vi "Main-OpenByFileVersionLabVIEW.vi"() -> ()   [LabVIEW 2017]
uses:
  States.ctl
  <vilib>/Utility/sysdir.llb/System Directory Type.ctl
  C:/Windows/System32/user32.dll
panel:
  in  "Simulation File Path":path
  in  "Simulation?":bool
  out "File Name & Version":string
  # "File :\nLabVIEW Version :\n\n\nAuthor :\nWebsite :"
  # "Ajay\nhttps://www.digiajay.com/"
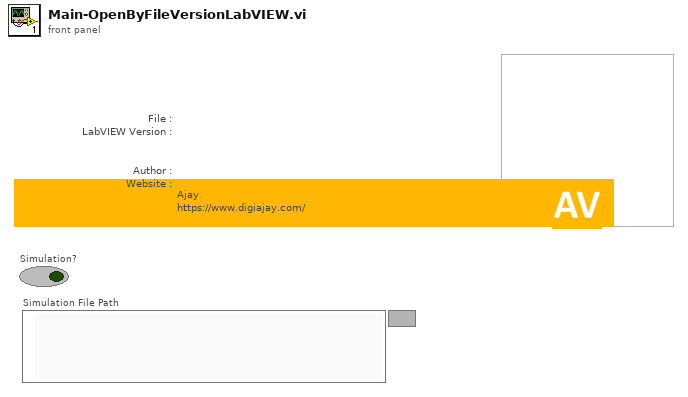
[diagram p1: front panel]
types:
  T1 = cluster{"File Path":path, "File LV Version":string, "File LV Exe Path":path, "Latest LV Exe Path":path, "Timeout Counter":i32, "NI Apps Folder":path, "Open x64 Bit?":bool, "Process Handle":refnum<k24>}
  T2 = typedef "States.ctl" = enum16{"Show FP", "Get LV Version & Path", "Update FP", "Get NI App Folder", "Get File LV Exe Path", "Get Latest LV Exe Path", "Open File Version LV", "Poll", "Exit"}
  T3 = enum32{"Invalid", "Standard", "Closed", "Hidden", "Minimized", "Maximized"}
  T4 = typedef "System Directory Type.ctl" = i32
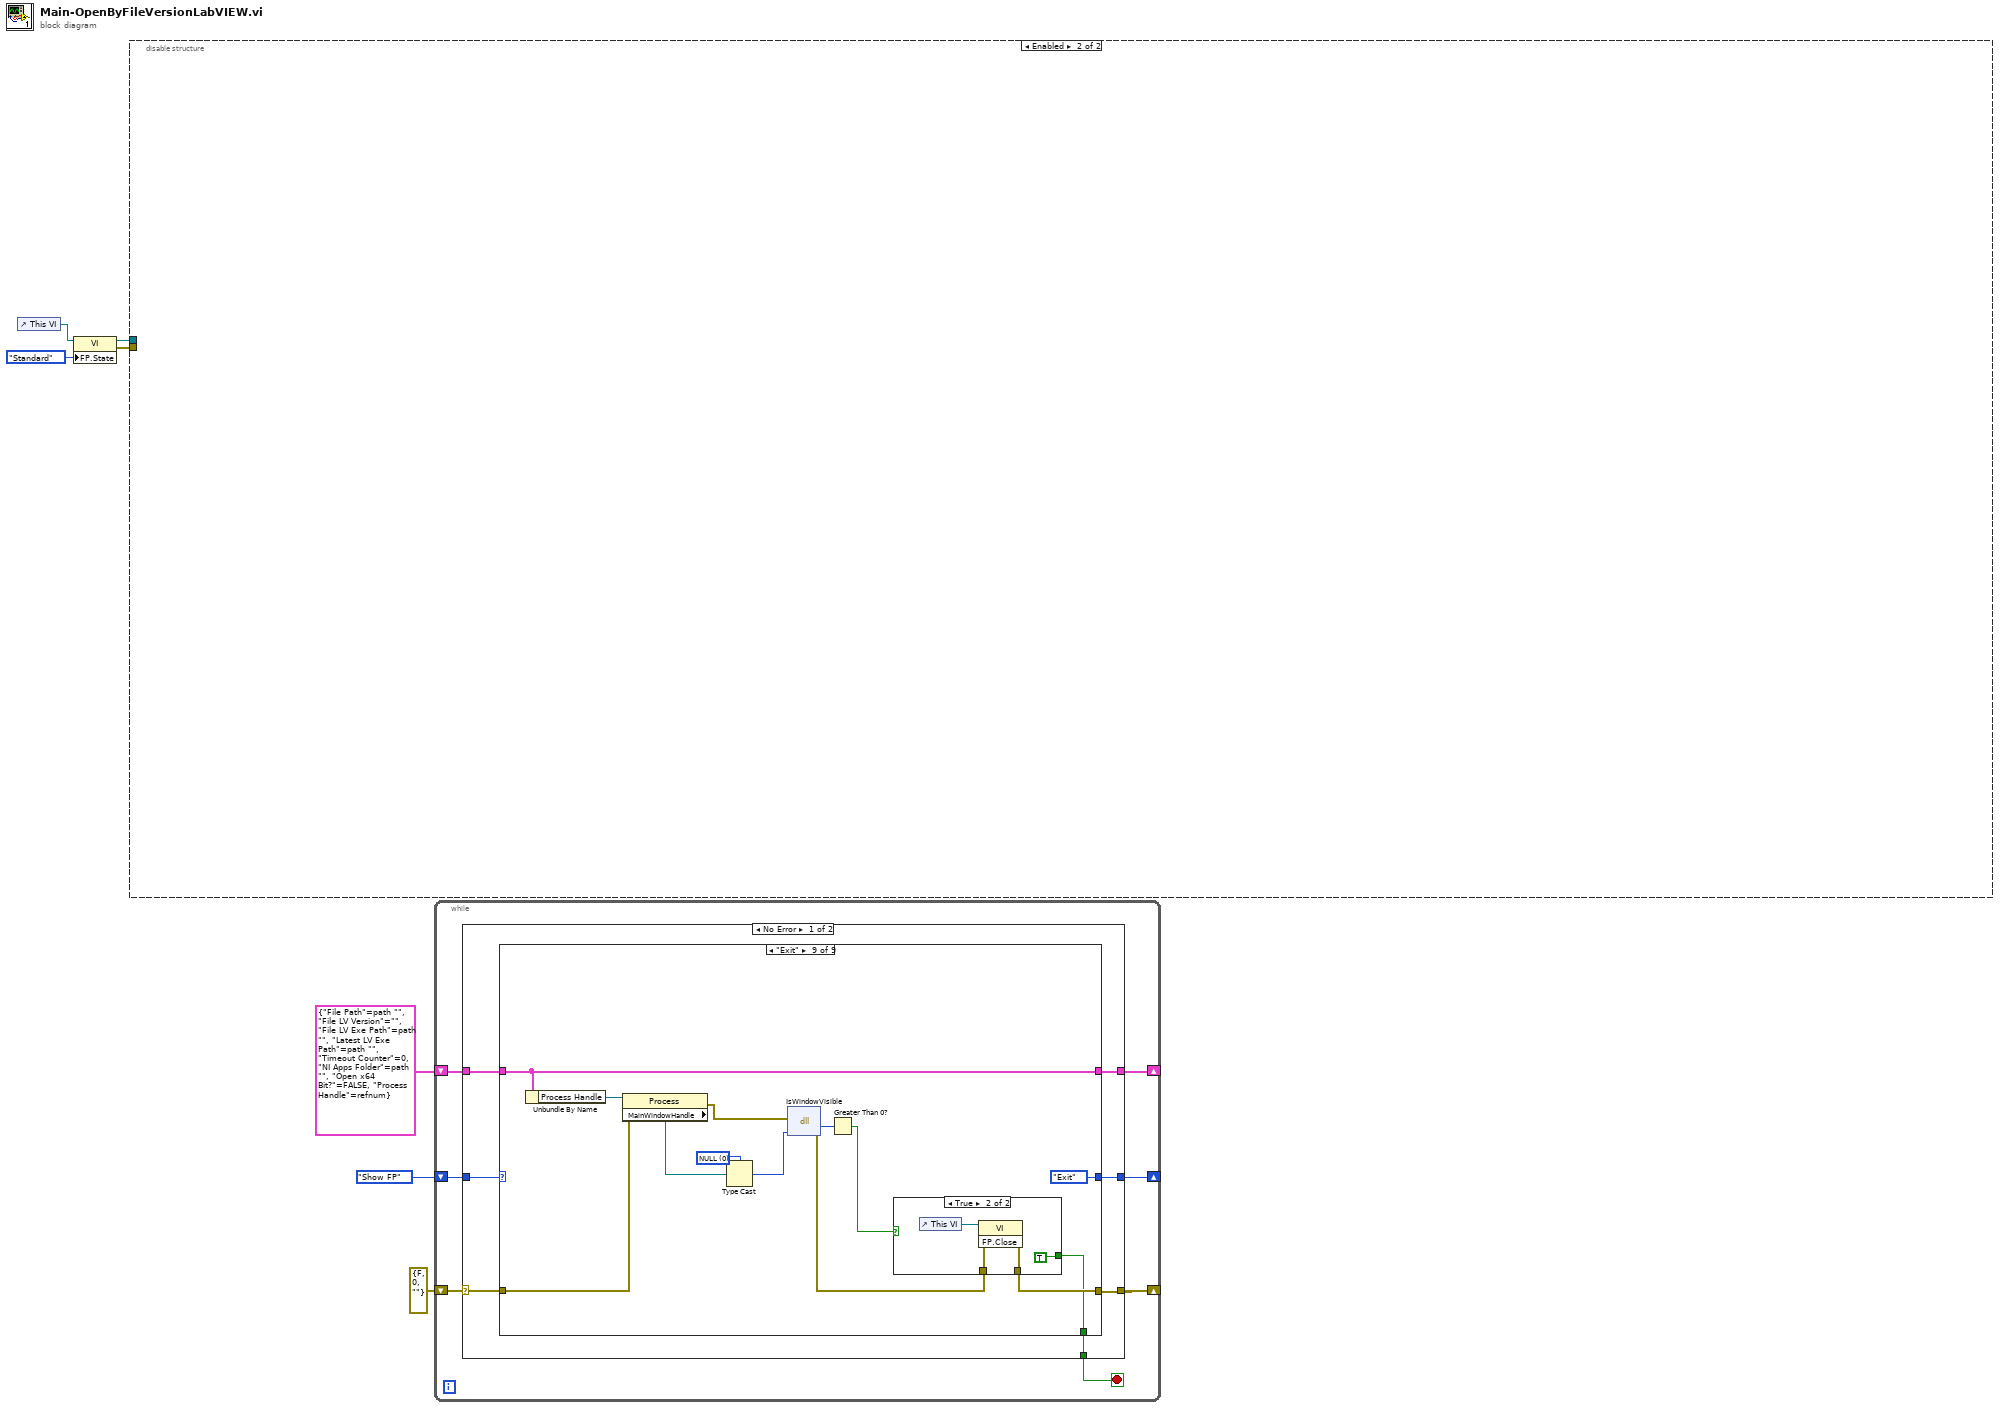
[diagram p0: block diagram]
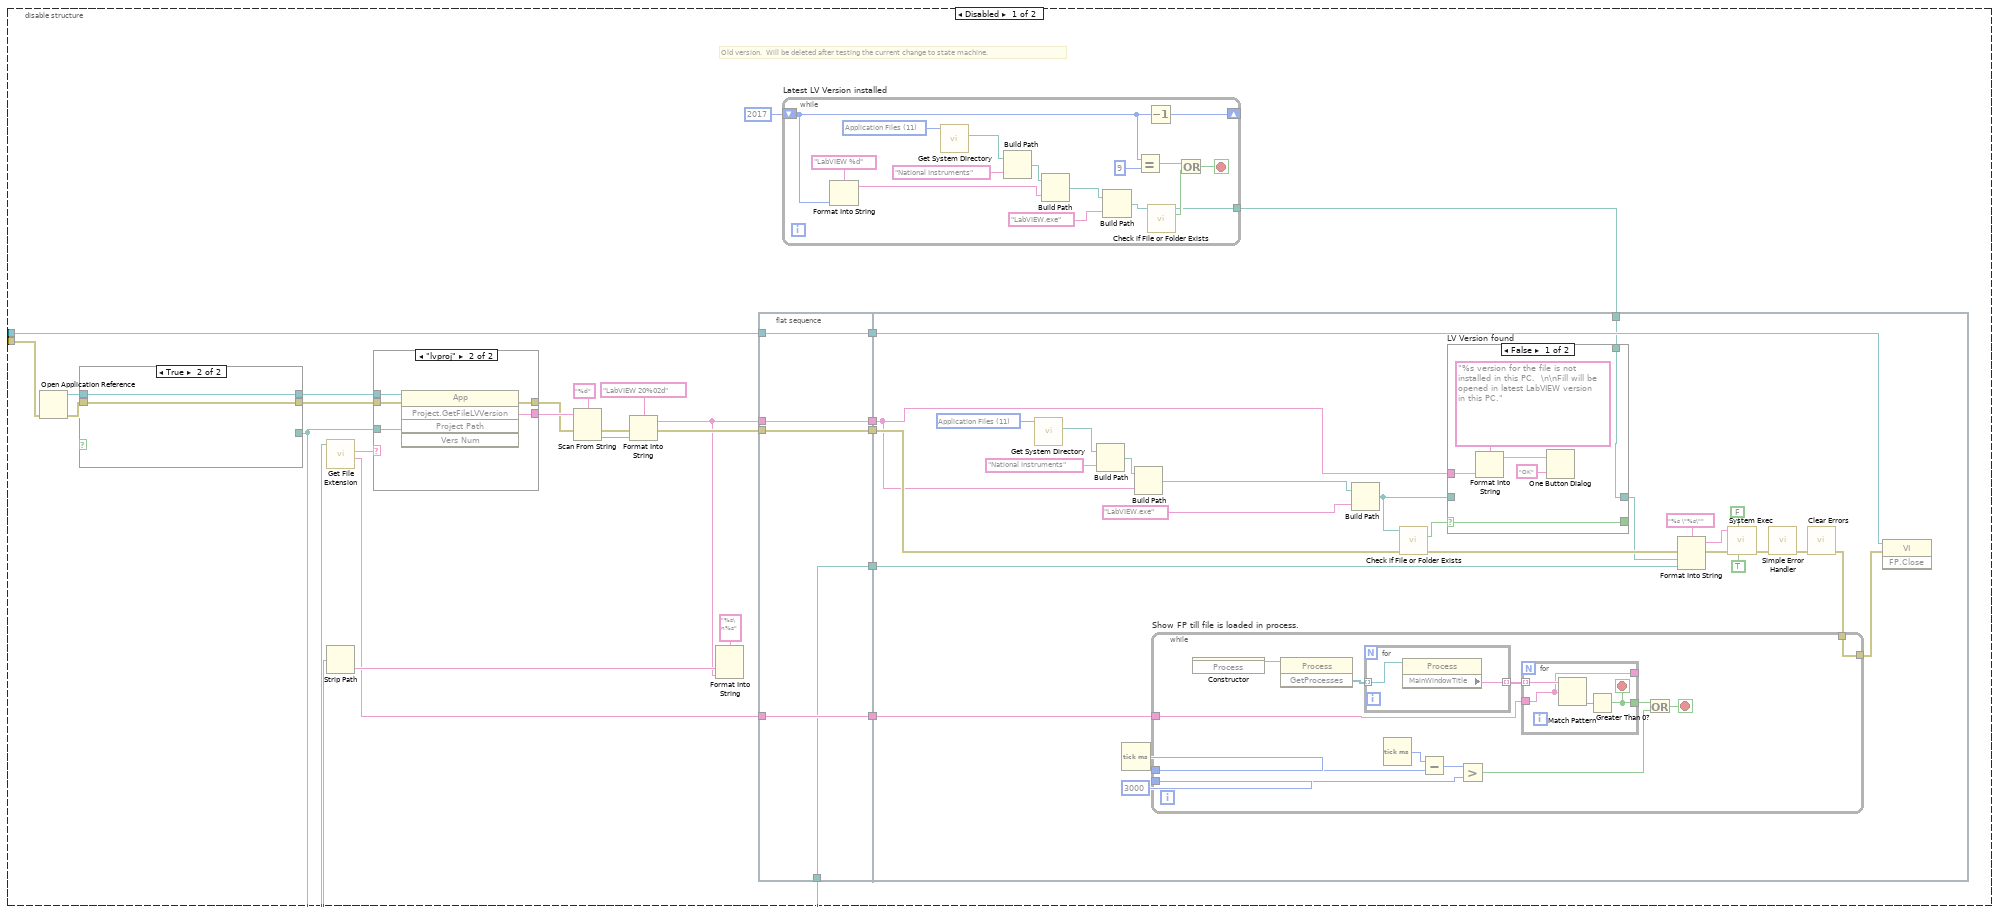
[diagram p2: hidden frame]
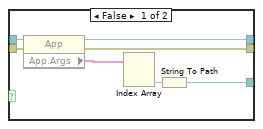
[diagram p4: hidden frame]
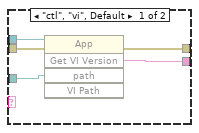
[diagram p5: hidden frame]
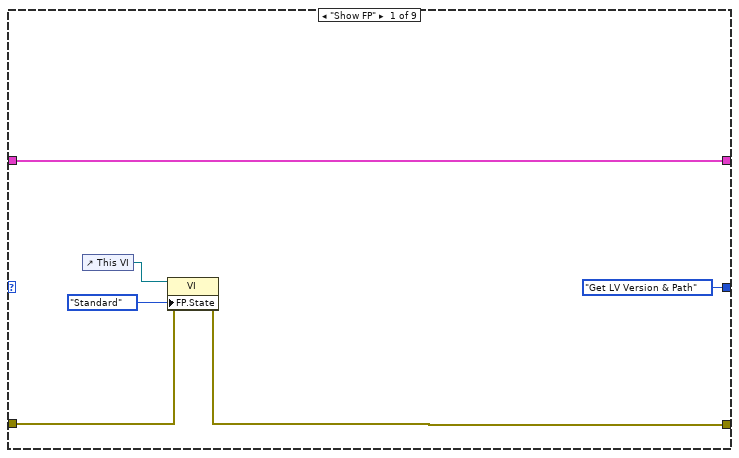
[diagram p6: hidden frame]
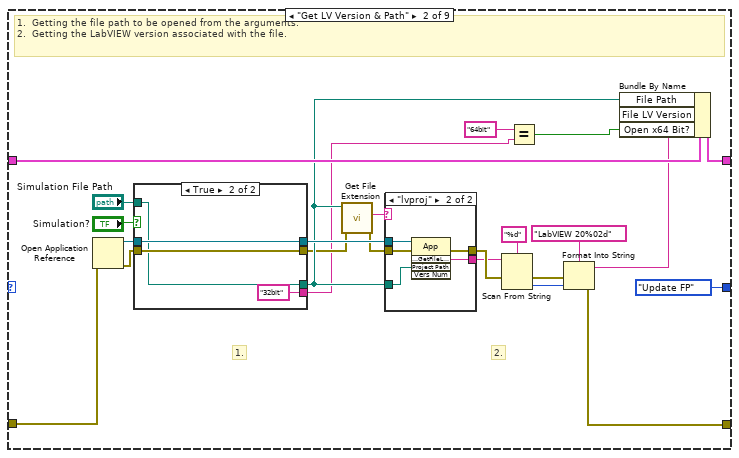
[diagram p7: hidden frame]
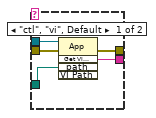
[diagram p8: hidden frame]
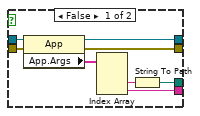
[diagram p9: hidden frame]
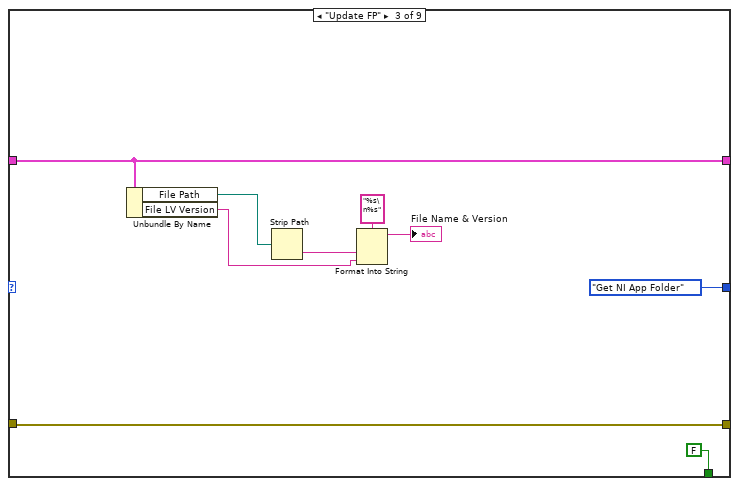
[diagram p10: hidden frame]
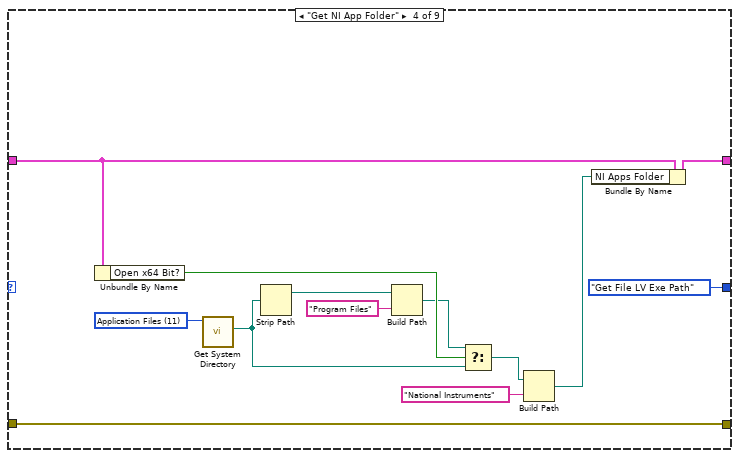
[diagram p11: hidden frame]
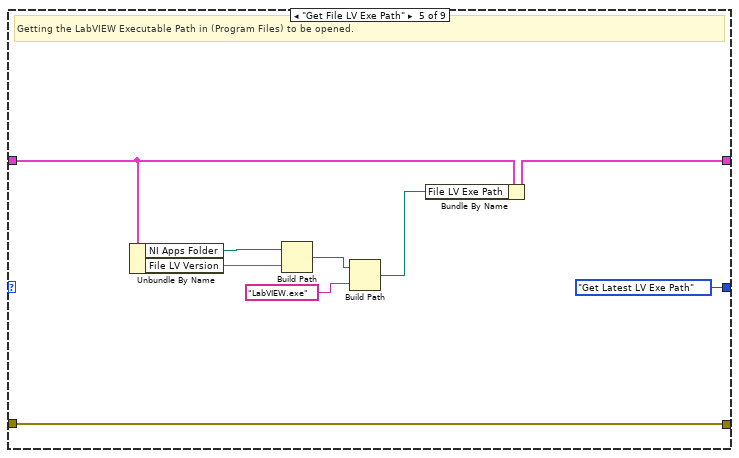
[diagram p12: hidden frame]
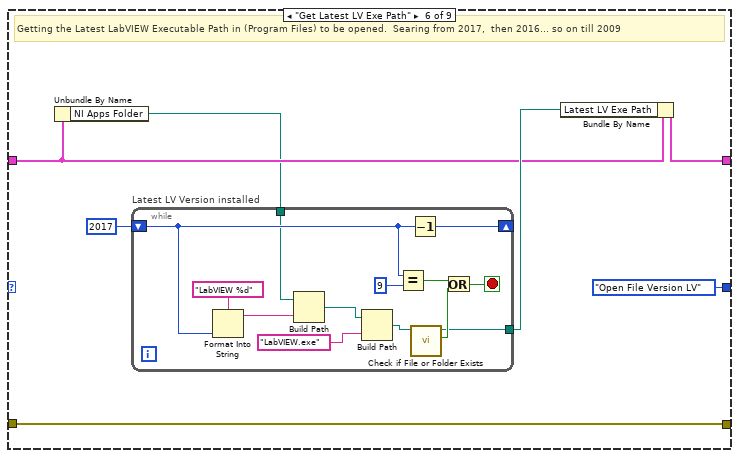
[diagram p13: hidden frame]
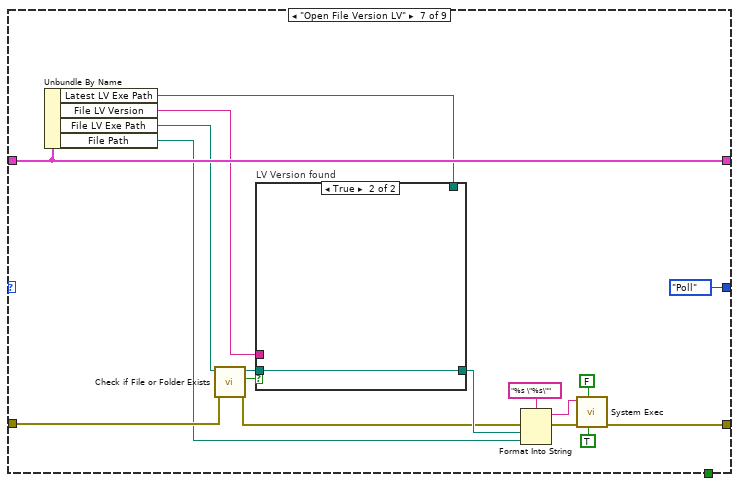
[diagram p14: hidden frame]
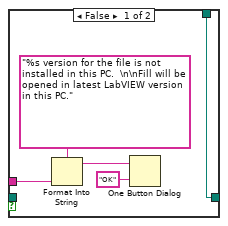
[diagram p15: hidden frame]
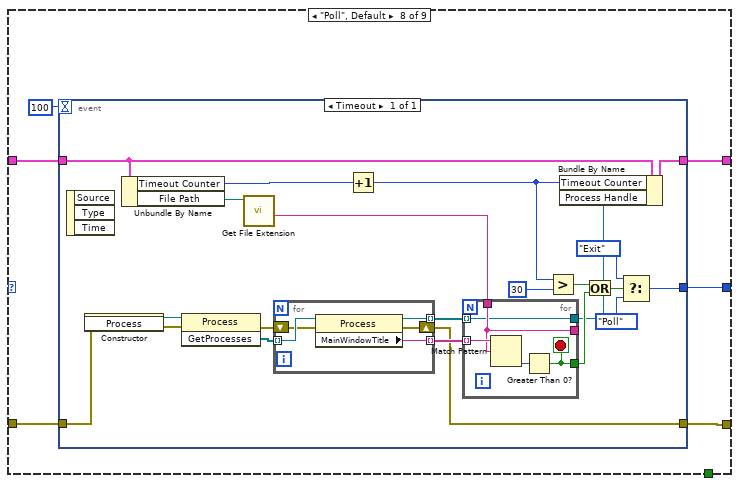
[diagram p16: hidden frame]
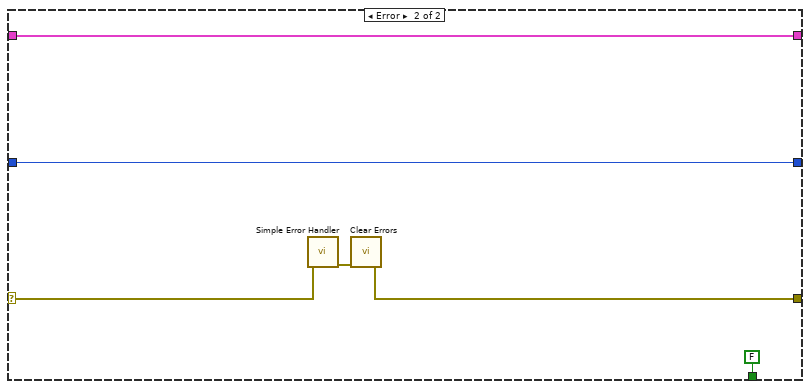
[diagram p18: hidden frame]
diagram:
  n1 = control-ref of="This VI"() -> (w7:refnum<vi>)
  n2 = property class="VI"(reference=w7, "FP.State"=T3."Standard" ("Front Panel Window:State")) -> (reference out=w5:refnum<vi>, error out=w4:errorcluster)  [unwired: 1 in]
  n3 = disable-structure shown="Enabled" {
    disable-tunnel: w5 -> [w19 _]
    disable-tunnel: w4 -> [w18 _]
    frame Disabled {
      # "Old version.  Will be deleted after testing the current change to state machine."
      n4 = Open Application Reference(8:w18) -> (0:w9:errorcluster, 3:w10:refnum<vi>)  [unwired: 3 in]
      n5 = case shown="True" {
        selector: _ -> [_ _]
        tunnel: [w98 w99] -> w28
        tunnel: [w97 w100] -> w27
        tunnel: [w96 _] -> w8
        tunnel: w10 -> [w95 w99]
        tunnel: w9 -> [w92 w100]
        frame False {
          n6 = property class="App"(reference=w95, error in=w92) -> (reference out=w98:refnum<vi>, error out=w97:errorcluster, "App.Args"=w94:string[])
          n7 = Index Array(array=w94) -> (element #2=w93:string)  [unwired: 2 in, 1 out]
          n8 = String To Path(string=w93) -> (path=w96:path)
        }
        frame True {
        }
      }
      n9 = call <vilib>:"Get File Extension.vi"("file"=w8) -> ("filename without extension"=w15:string, "lowercase file extension"=w20:string)  [unwired: 6 in, 3 out]
      n10 = Strip Path(path=w8) -> (name=w17:string)  [unwired: 1 out]
      n11 = case shown="\"lvproj\"" w20 {
        tunnel: w28 -> [w121 w126]
        tunnel: w27 -> [w120 w125]
        tunnel: [w119 w124] -> w26
        tunnel: [w118 w123] -> w24
        tunnel: w8 -> [w117 w122]
        frame "ctl", "vi", Default {
          n12 = invoke class="App" method="Get VI Version"(reference=w121, error in=w120, "path"=w117) -> (error out=w118:errorcluster, "GetVIVers"=w119:string)  [unwired: 2 in, 3 out]
        }
        frame "lvproj" {
          n13 = invoke class="App" method="Project.GetFileLVVersion"(reference=w126, error in=w125, "Project Path"=w122) -> (error out=w123:errorcluster, "Project.GetFileLVVersion"=w124:string)  [unwired: 2 in, 3 out]
        }
      }
      n14 = Scan From String(format string="%d", input string=w26, error in=w24) -> (error out=w21:errorcluster, output 1=w23:i32)  [unwired: 2 in, 2 out]
      n15 = Format Into String(format string="LabVIEW 20%02d", error in=w21, w23) -> (resulting string=w13:string, error out=w14:errorcluster)  [unwired: 1 in]
      n16 = Format Into String(format string="%s\n%s", w17, w13) -> ()  [unwired: 2 in, 2 out]
      n17 = flat-sequence {
        tunnel: w13 -> [w35]
        tunnel: w14 -> [w36]
        tunnel: w15 -> [w37]
        tunnel: w19 -> [w38]
        tunnel: [w38] -> w33
        tunnel: [w34] -> w32
        tunnel: [w37] -> w31
        tunnel: [w36] -> w30
        tunnel: [w35] -> w29
        tunnel: w8 -> [w34]
        tunnel: w11 -> [w39]
        tunnel: w33 -> [w59]
        tunnel: w32 -> [w58]
        tunnel: w31 -> [w53]
        tunnel: w30 -> [w51]
        tunnel: w29 -> [w42]
        frame #0 {
        }
        frame #1 {
          w65 = T4 11 items=["User Home"=0, "User Desktop"=1, "User Documents"=2, "User Application Data"=3, "User Preferences"=4, "User Temporary"=5, "Public Documents"=6, "Public Application Data"=7, "Public Preferences"=8, "Public Cache"=13, "System Core Libraries"=9, "System Installed Libraries"=10, "Application Files"=11, "Boot Volume Root"=12] ("system directory type")
          n18 = call <vilib>:"Get System Directory.vi"("system directory type"=w65) -> ("system directory"=w64:path)  [unwired: 10 in]
          n19 = Build Path(base path=w64, name or relative path="National Instruments") -> (appended path=w62:path)
          n20 = Tick Count (ms)() -> (millisecond timer value=w57:u32)
          n21 = Build Path(base path=w62, name or relative path=w42) -> (appended path=w61:path)
          n22 = Build Path(base path=w61, name or relative path="LabVIEW.exe") -> (appended path=w41:path)
          n23 = call <vilib>:"Check if File or Folder Exists.vi"("error in (no error)"=w51, "path"=w41) -> ("error out"=w50:errorcluster, "file or folder exists?"=w44:bool)  [unwired: 7 in, 1 out]
          n24 = case "LV Version found" shown="False" w44 {
            selector: w44 -> [w69 w73]
            tunnel: [w69 w73] -> _
            tunnel: w42 -> [w67 _]
            tunnel: [w66 w72] -> w43
            tunnel: w41 -> [_ w72]
            tunnel: w39 -> [w66 _]
            frame False {
              n25 = Format Into String(format string="%s version for the file is not installed in this PC.  \n\nFill will be opened in latest LabVIEW version in this PC." ("message"), w67) -> (resulting string=w68:string)  [unwired: 2 in, 1 out]
              n26 = One Button Dialog(message=w68, button name ("OK")="OK") -> ()  [unwired: 1 out]
            }
            frame True {
            }
          }
          n27 = Format Into String(format string="%s \"%s\"" ("command line"), error in=w50, w43, w58) -> (resulting string=w48:string, error out=w47:errorcluster)  [unwired: 1 in]
          n28 = call <vilib>:"System Exec.vi"("run minimized? (F)"=TRUE, "wait until completion? (T)"=FALSE, "error in (no error)"=w47, "command line"=w48) -> ("error out"=w54:errorcluster)  [unwired: 4 in, 3 out]
          n29 = call <vilib>:"Simple Error Handler.vi"("error in (no error)"=w54) -> ("error out"=w60:errorcluster)  [unwired: 4 in, 4 out]
          n30 = call <vilib>:"Clear Errors.vi"("error in (no error)"=w60) -> ("error out"=w52:errorcluster)  [unwired: 5 in, 1 out]
          n31 = while "Show FP till file is loaded in process." {
            tunnel: w57 -> [w82]
            tunnel: u32 3000 ("y") -> [w80]
            tunnel: [w78] -> w55
            tunnel: w52 -> [w78]
            tunnel: w53 -> [w77]
            stop <- w84 stop-if-true
            n32 = constructor class="Process"() -> (reference out=w75:refnum<k24>)  [unwired: 3 in, 2 out]
            n33 = invoke class="Process" method="GetProcesses"(reference=w75) -> ("GetProcesses"=w74:refnum<k24>[])  [unwired: 2 in, 2 out]
            n34 = for {
              tunnel: w74 -> [w91] mode=indexing
              tunnel: [w90] -> w85 mode=indexing
              n35 = property class="Process"(reference=w91) -> ("MainWindowTitle"=w90:string)  [unwired: 1 in, 2 out]
            }
            n36 = Tick Count (ms)() -> (millisecond timer value=w83:u32)
            n37 = Subtract(x=w83, y=w82) -> (x-y=w81:u32)
            n38 = Greater?(x=w81, y=w80) -> (0:w79:bool)
            n39 = for {
              tunnel: w85 -> [w89] mode=indexing
              tunnel: [w87] -> w76
              tunnel: w77 -> [w86]
              tunnel: [w86] -> _
              stop <- w87 stop-if-true
              n40 = Match Pattern(string=w89, regular expression=w86) -> (offset past match=w88:i32)  [unwired: 1 in, 3 out]
              n41 = Greater Than 0?(x=w88) -> (x > 0?=w87:bool)
            }
            n42 = Or(x=w76, y=w79) -> (x .or. y?=w84:bool)
          }
          n43 = invoke class="VI" method="FP.Close"(reference=w59, error in=w55) -> ()  [unwired: 1 in, 3 out]
        }
      }
      n44 = while "Latest LV Version installed" {
        shift-right: [w106] -> _
        shift-left: 2017 ("input 1") -> [w105]
        tunnel: [w101] -> w11
        stop <- w103 stop-if-true
        w110 = T4 11 items=["User Home"=0, "User Desktop"=1, "User Documents"=2, "User Application Data"=3, "User Preferences"=4, "User Temporary"=5, "Public Documents"=6, "Public Application Data"=7, "Public Preferences"=8, "Public Cache"=13, "System Core Libraries"=9, "System Installed Libraries"=10, "Application Files"=11, "Boot Volume Root"=12] ("system directory type")
        n45 = Format Into String(format string="LabVIEW %d", w105) -> (resulting string=w109:string)  [unwired: 2 in, 1 out]
        n46 = call <vilib>:"Get System Directory.vi"("system directory type"=w110) -> ("system directory"=w111:path)  [unwired: 10 in]
        n47 = Build Path(base path=w111, name or relative path="National Instruments") -> (appended path=w113:path)
        n48 = Build Path(base path=w113, name or relative path=w109) -> (appended path=w114:path)
        n49 = Build Path(base path=w114, name or relative path="LabVIEW.exe") -> (appended path=w108:path)
        n50 = Equal?(x=w105, y=9) -> (x = y?=w102:bool)
        n51 = Decrement(x=w105) -> (x-1=w106:i32)
        n52 = call <vilib>:"Check if File or Folder Exists.vi"("path"=w108) -> ("file or folder exists?"=w107:bool, "dup path"=w101:path)  [unwired: 8 in, 1 out]
        n53 = Or(x=w102, y=w107) -> (x .or. y?=w103:bool)
      }
    }
    frame Enabled {
    }
  }
  n54 = while {
    shift-right: [w132] -> _
    shift-left: errorcluster {"status"=FALSE, "code"=0, "source"=""} ("error out") -> [w131]
    shift-right: [w129] -> _
    shift-left: T1 {"File Path"=path "", "File LV Version"="", "File LV Exe Path"=path "", "Latest LV Exe Path"=path "", "Timeout Counter"=0, "NI Apps Folder"=path "", "Open x64 Bit?"=FALSE, "Process Handle"=refnum} -> [w130]
    shift-right: [w128] -> _
    shift-left: States."Show FP" -> [w133]
    stop <- w127 stop-if-true
    n55 = case shown="No Error" w131 {
      selector: w131 -> [w138 w327]
      tunnel: w133 -> [w140 w325]
      tunnel: [w139 w326] -> w132
      tunnel: w130 -> [w137 w324]
      tunnel: [w136 w324] -> w129
      tunnel: [w135 w325] -> w128
      tunnel: [w134 FALSE] -> w127
      frame No Error {
        n56 = case shown="\"Exit\"" w140 {
          tunnel: [w141 w152 w201 w214 w223 w230 w248 w269 w317] -> w139
          tunnel: w138 -> [w144 w166 w201 w214 w223 w230 w249 w268 w314]
          tunnel: w137 -> [w143 w167 w198 w210 w220 w225 w252 w270 w316]
          tunnel: [w143 w165 w198 w211 w218 w228 w252 w271 w316] -> w136
          tunnel: [States."Get LV Version & Path" States."Update FP" States."Get NI App Folder" States."Get File LV Exe Path" States."Get Latest LV Exe Path" States."Open File Version LV" States."Poll" w267 States."Exit"] -> w135
          tunnel: [_ _ FALSE _ _ _ _ _ w310] -> w134
          frame "Show FP" {
            n57 = control-ref of="This VI"() -> (w145:refnum<vi>)
            n58 = property class="VI"(reference=w145, error in=w144, "FP.State"=T3."Standard" ("Front Panel Window:State")) -> (error out=w141:errorcluster)  [unwired: 1 out]
          }
          frame "Get LV Version & Path" {
            # "2."
            # "1."
            # "1.  Getting the file path to be opened from the arguments.\n2.  Getting the LabVIEW version associated with the file."
            n59 = Open Application Reference(8:w166) -> (0:w170:errorcluster, 3:w169:refnum<vi>)  [unwired: 3 in]
            n60 = case shown="True" "Simulation?" {
              tunnel: [w188 w191] -> w156
              tunnel: [w187 w192] -> w154
              tunnel: [w186 w190] -> w155
              tunnel: w169 -> [w185 w191]
              tunnel: w170 -> [w182 w192]
              tunnel: "Simulation File Path" -> [_ w190]
              tunnel: [w181 "32bit"] -> w148
              frame False {
                n61 = property class="App"(reference=w185, error in=w182) -> (reference out=w188:refnum<vi>, error out=w187:errorcluster, "App.Args"=w184:string[])
                n62 = Index Array(array=w184) -> (element #2=w183:string, element #3=w181:string)  [unwired: 3 in, 1 out]
                n63 = String To Path(string=w183) -> (path=w186:path)
              }
              frame True {
              }
            }
            n64 = call <vilib>:"Get File Extension.vi"("error in (no error)"=w154, "file"=w155) -> ("error out"=w153:errorcluster, "lowercase file extension"=w163:string)  [unwired: 5 in, 3 out]
            n65 = case shown="\"lvproj\"" w163 {
              tunnel: w156 -> [w175 w180]
              tunnel: w153 -> [w174 w179]
              tunnel: [w173 w178] -> w157
              tunnel: [w172 w177] -> w159
              tunnel: w155 -> [w171 w176]
              frame "ctl", "vi", Default {
                n66 = invoke class="App" method="Get VI Version"(reference=w175, error in=w174, "path"=w171) -> (error out=w172:errorcluster, "GetVIVers"=w173:string)  [unwired: 2 in, 3 out]
              }
              frame "lvproj" {
                n67 = invoke class="App" method="Project.GetFileLVVersion"(reference=w180, error in=w179, "Project Path"=w176) -> (error out=w177:errorcluster, "Project.GetFileLVVersion"=w178:string)  [unwired: 2 in, 3 out]
              }
            }
            n68 = Scan From String(format string="%d", input string=w157, error in=w159) -> (error out=w162:errorcluster, output 1=w160:i32)  [unwired: 2 in, 2 out]
            n69 = Equal?(x="64bit", y=w148) -> (x = y?=w149:bool)
            n70 = Format Into String(format string="LabVIEW 20%02d", error in=w162, w160) -> (resulting string=w151:string, error out=w152:errorcluster)  [unwired: 1 in]
            n71 = Bundle By Name(cluster=w167, "File Path"=w155, "File LV Version"=w151, "Open x64 Bit?"=w149) -> (w165:T1)
          }
          frame "Update FP" {
            n72 = Unbundle By Name(w198) -> ("File Path"=w197:path, "File LV Version"=w195:string)
            n73 = Strip Path(path=w197) -> (name=w196:string)  [unwired: 1 out]
            n74 = Format Into String(format string="%s\n%s", w196, w195) -> (resulting string=→"File Name & Version":string)  [unwired: 2 in, 1 out]
          }
          frame "Get NI App Folder" {
            w213 = T4 11 items=["User Home"=0, "User Desktop"=1, "User Documents"=2, "User Application Data"=3, "User Preferences"=4, "User Temporary"=5, "Public Documents"=6, "Public Application Data"=7, "Public Preferences"=8, "Public Cache"=13, "System Core Libraries"=9, "System Installed Libraries"=10, "Application Files"=11, "Boot Volume Root"=12] ("system directory type")
            n75 = Unbundle By Name(w210) -> ("Open x64 Bit?"=w209:bool)
            n76 = call <vilib>:"Get System Directory.vi"("system directory type"=w213) -> ("system directory"=w206:path)  [unwired: 10 in]
            n77 = Strip Path(path=w206) -> (stripped path=w208:path)  [unwired: 1 out]
            n78 = Build Path(base path=w208, name or relative path="Program Files") -> (appended path=w205:path)
            n79 = Select(t=w205, s=w209, f=w206) -> (s? t:f=w204:path)
            n80 = Build Path(base path=w204, name or relative path="National Instruments") -> (appended path=w203:path)
            n81 = Bundle By Name(cluster=w210, "NI Apps Folder"=w203) -> (w211:T1)
          }
          frame "Get File LV Exe Path" {
            # "Getting the LabVIEW Executable Path in (Program Files) to be opened."
            n82 = Unbundle By Name(w220) -> ("NI Apps Folder"=w215:path, "File LV Version"=w219:string)
            n83 = Build Path(base path=w215, name or relative path=w219) -> (appended path=w221:path)
            n84 = Build Path(base path=w221, name or relative path="LabVIEW.exe") -> (appended path=w217:path)
            n85 = Bundle By Name(cluster=w220, "File LV Exe Path"=w217) -> (w218:T1)
          }
          frame "Get Latest LV Exe Path" {
            # "Getting the Latest LabVIEW Executable Path in (Program Files) to be opened.  Searing from 2017,  then 2016... so on till 2009"
            n86 = Unbundle By Name(w225) -> ("NI Apps Folder"=w224:path)
            n87 = while "Latest LV Version installed" {
              shift-right: [w237] -> _
              shift-left: 2017 ("input 1") -> [w236]
              tunnel: [w232] -> w227
              tunnel: w224 -> [w231]
              stop <- w234 stop-if-true
              n88 = Format Into String(format string="LabVIEW %d", w236) -> (resulting string=w240:string)  [unwired: 2 in, 1 out]
              n89 = Build Path(base path=w231, name or relative path=w240) -> (appended path=w241:path)
              n90 = Build Path(base path=w241, name or relative path="LabVIEW.exe") -> (appended path=w239:path)
              n91 = Equal?(x=w236, y=9) -> (x = y?=w233:bool)
              n92 = Decrement(x=w236) -> (x-1=w237:i32)
              n93 = call <vilib>:"Check if File or Folder Exists.vi"("path"=w239) -> ("file or folder exists?"=w238:bool, "dup path"=w232:path)  [unwired: 8 in, 1 out]
              n94 = Or(x=w233, y=w238) -> (x .or. y?=w234:bool)
            }
            n95 = Bundle By Name(cluster=w225, "Latest LV Exe Path"=w227) -> (w228:T1)
          }
          frame "Open File Version LV" {
            n96 = Unbundle By Name(w252) -> ("Latest LV Exe Path"=w247:path, "File LV Version"=w250:string, "File LV Exe Path"=w251:path, "File Path"=w245:path)
            n97 = call <vilib>:"Check if File or Folder Exists.vi"("error in (no error)"=w249, "path"=w251) -> ("error out"=w253:errorcluster, "file or folder exists?"=w259:bool, "dup path"=w246:path)  [unwired: 7 in]
            n98 = case "LV Version found" shown="True" w259 {
              tunnel: w250 -> [w262 _]
              tunnel: [w261 w266] -> w260
              tunnel: w246 -> [_ w266]
              tunnel: w247 -> [w261 _]
              frame False {
                n99 = Format Into String(format string="%s version for the file is not installed in this PC.  \n\nFill will be opened in latest LabVIEW version in this PC." ("message"), w262) -> (resulting string=w263:string)  [unwired: 2 in, 1 out]
                n100 = One Button Dialog(message=w263, button name ("OK")="OK") -> ()  [unwired: 1 out]
              }
              frame True {
              }
            }
            n101 = Format Into String(format string="%s \"%s\"" ("command line"), error in=w253, w260, w245) -> (resulting string=w255:string, error out=w256:errorcluster)  [unwired: 1 in]
            n102 = call <vilib>:"System Exec.vi"("run minimized? (F)"=TRUE, "wait until completion? (T)"=FALSE, "error in (no error)"=w256, "command line"=w255) -> ("error out"=w248:errorcluster)  [unwired: 4 in, 3 out]
          }
          frame "Poll", Default {
            n103 = event shown="[0] Timeout" {
              selector: _ -> [_]
              dyn-events: _ -> [_]
              timeout: 100 -> [_]
              tunnel: [w287] -> w271
              tunnel: w270 -> [w290]
              tunnel: [w279] -> w269
              tunnel: w268 -> [w281]
              tunnel: [w276] -> w267
              event Timeout {
                n104 = event-data() -> ()  [unwired: 1 in, 3 out]
                n105 = constructor class="Process"(error in=w281) -> (reference out=w293:refnum<k24>, error out=w282:errorcluster)  [unwired: 2 in, 1 out]
                n106 = Unbundle By Name(w290) -> ("Timeout Counter"=w286:i32, "File Path"=w289:path)
                n107 = invoke class="Process" method="GetProcesses"(reference=w293, error in=w282) -> (error out=w280:errorcluster, "GetProcesses"=w294:refnum<k24>[])  [unwired: 1 in, 1 out]
                n108 = call <vilib>:"Get File Extension.vi"("file"=w289) -> ("filename without extension"=w288:string)  [unwired: 6 in, 4 out]
                n109 = for {
                  tunnel: w294 -> [w304] mode=indexing
                  tunnel: [w303] -> w291 mode=indexing
                  shift-right: [w302] -> w279
                  shift-left: w280 -> [w301]
                  tunnel: [w300] -> w274 mode=indexing
                  n110 = property class="Process"(reference=w304, error in=w301) -> (reference out=w300:refnum<k24>, error out=w302:errorcluster, "MainWindowTitle"=w303:string)
                }
                n111 = Increment(x=w286) -> (x+1=w285:i32)
                n112 = for {
                  tunnel: w291 -> [w299] mode=indexing
                  tunnel: [w297] -> w292
                  tunnel: w288 -> [w296]
                  tunnel: [w296] -> _
                  tunnel: w274 -> [w295] mode=indexing
                  tunnel: [w295] -> w273
                  stop <- w297 stop-if-true
                  n113 = Match Pattern(string=w299, regular expression=w296) -> (offset past match=w298:i32)  [unwired: 1 in, 3 out]
                  n114 = Greater Than 0?(x=w298) -> (x > 0?=w297:bool)
                }
                n115 = Greater?(x=w285, y=30) -> (0:w283:bool)
                n116 = Bundle By Name(cluster=w290, "Timeout Counter"=w285, "Process Handle"=w273) -> (w287:T1)
                n117 = Or(x=w283, y=w292) -> (x .or. y?=w278:bool)
                n118 = Select(t=States."Exit", s=w278, f=States."Poll") -> (s? t:f=w276:T2)
              }
            }
          }
          frame "Exit" {
            w308 = u32 0 items=["NULL"]
            n119 = Unbundle By Name(w316) -> ("Process Handle"=w315:refnum<k24>)
            n120 = property class="Process"(reference=w315, error in=w314) -> (error out=w307:errorcluster, "MainWindowHandle"=w306:refnum<k24>)  [unwired: 1 out]
            n121 = Type Cast(type=w308, x=w306) -> (*(type *) &x=w305:u32)
            n122 = dll-call lib="C:/Windows/System32/user32.dll" fn="IsWindowVisible"(error in=w307, "WindowHandle"=w305) -> (error out=w313:errorcluster, "ReturnVisible"=w312:i32)  [unwired: 3 in, 1 out]
            n123 = Greater Than 0?(x=w312) -> (x > 0?=w311:bool)
            n124 = case shown="True" w311 {
              tunnel: w313 -> [w318 w321]
              tunnel: [w318 w320] -> w317
              tunnel: [_ TRUE] -> w310
              frame False {
              }
              frame True {
                n125 = control-ref of="This VI"() -> (w322:refnum<vi>)
                n126 = invoke class="VI" method="FP.Close"(reference=w322, error in=w321) -> (error out=w320:errorcluster)  [unwired: 1 in, 2 out]
              }
            }
          }
        }
      }
      frame Error {
        n127 = call <vilib>:"Simple Error Handler.vi"("error in (no error)"=w327) -> ("error out"=w328:errorcluster)  [unwired: 4 in, 4 out]
        n128 = call <vilib>:"Clear Errors.vi"("error in (no error)"=w328) -> ("error out"=w326:errorcluster)  [unwired: 5 in, 1 out]
      }
    }
  }
